vi "Forward Acknowledgement.vi"(8 "error in (no error)":errorcluster, 10 "Acknowledgement":refnum<class "Ack.lvclass">, 11 "MQTT Server":refnum<class "Server.lvclass">) -> (0 "error out":errorcluster, 3 "MQTT Server":refnum<class "Server.lvclass">)   [LabVIEW 2013, in "MQTT Server.lvlib" / "Server.lvclass"]
uses:
  Server.lvclass
  <vilib>/LabVIEW Open Source Project/MQTT Control Packets/Control Packets/Ack/Ack.lvclass
  Server.lvclass/Server.ctl
  <vilib>/LabVIEW Open Source Project/MQTT Control Packets/Control Packets/PUBLISH/PUBLISH.lvclass
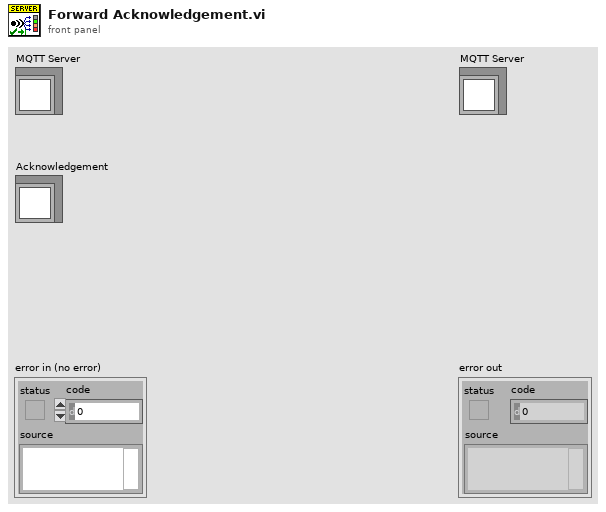
[diagram p1: front panel]
types:
  T1 = typedef "MQTT Server.lvlib/Server.lvclass/Private Events -- cluster.ctl" = cluster{"Inbound Packet":refnum<user-event>, "Inbound Ack":refnum<user-event>}
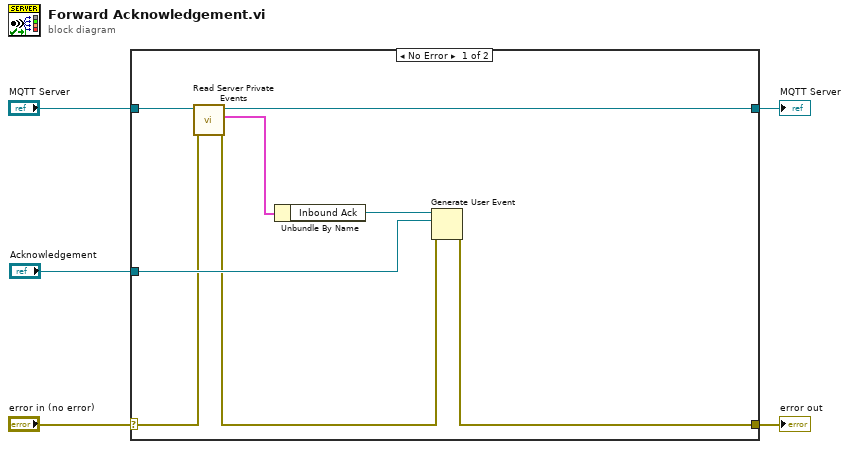
[diagram p0: block diagram]
diagram:
  n1 = case shown="No Error" "error in (no error)" {
    selector: "error in (no error)" -> [w7 w15]
    tunnel: [w13 w15] -> w4
    tunnel: [w10 w14] -> w2
    tunnel: "MQTT Server" -> [w9 w14]
    tunnel: "Acknowledgement" -> [w12 _]
    frame No Error {
      n2 = call "Read Server Private Events.vi"("error in (no error)"=w7, "Server in"=w9) -> ("error out"=w6:errorcluster, "Server Private Events"=w8:T1, "Server out"=w10:refnum<class "Server.lvclass">)  [unwired: 7 in]
      n3 = Unbundle By Name(w8) -> ("Inbound Ack"=w11:refnum<user-event>)
      n4 = Generate User Event(user event=w11, event data cluster=w12, error in=w6) -> (error out=w13:errorcluster)  [unwired: 1 in, 1 out]
    }
    frame Error {
    }
  }
  "error out" <- w4
  "MQTT Server" <- w2
